vi "Convert Grayscale Image to Binary Image LV2012 NIVerified.vi"() -> ()   [LabVIEW 2021, in "Test VIs.lvclass"]
doc: "This VI demonstrates how to convert a grayscale image into a binary image.\nTo do so, you can use the IMAQ Threshold function with a lower limit = 0 and upper limit = 1."
uses:
  Test VIs/Test VIs.lvclass
  <vilib>/vision/NI_Vision_Development_Module.lvlib
panel:
  in  "Range":cluster{"Lower value":sgl, "Upper value":sgl}={"Lower value"=100.0, "Upper value"=200.0}
  out "Original Image":T1(plugin-control)
  out "Binary Image":T1(plugin-control)
  # "Overview: Demonstrates how to convert a grayscale image into a binary image with the IMAQ Threshold VI. \nRequirements: LabVIEW Base Development System 2012 (or compatible)\n                            NI Vision Development Module 2012 (or compatible)\nInstructions: \n1. Run the VI.\n2. Select a grayscale image which should be converted to a binary image. An example image is already provided with this example."
  # "The palette for this Image Display need to be set to Binary, \notherwise no picture will be displayed.\nRight click on the image and select Palette >> Binary"
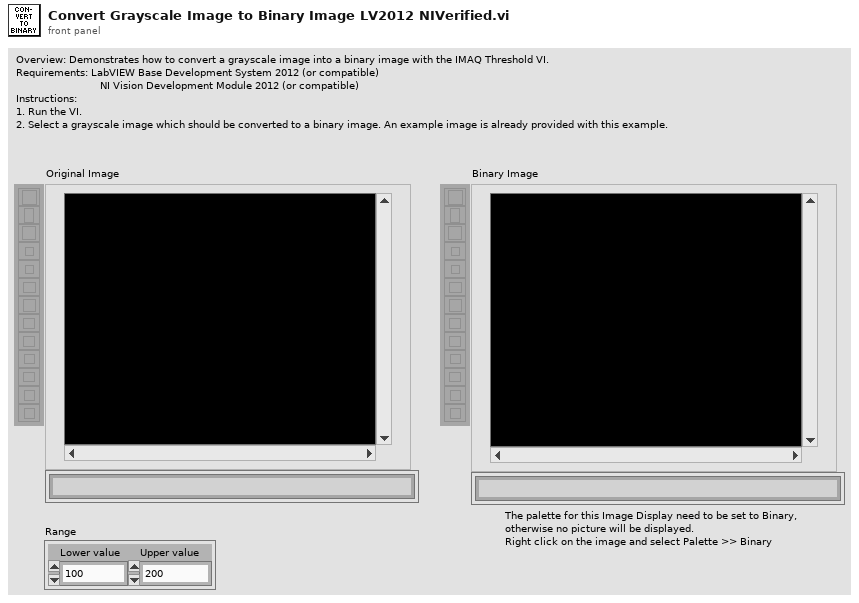
[diagram p1: front panel]
types:
  T1 = typedef "IMAQ Image.ctl" = refnum<image>
  T2 = typedef "Image Type" = u32
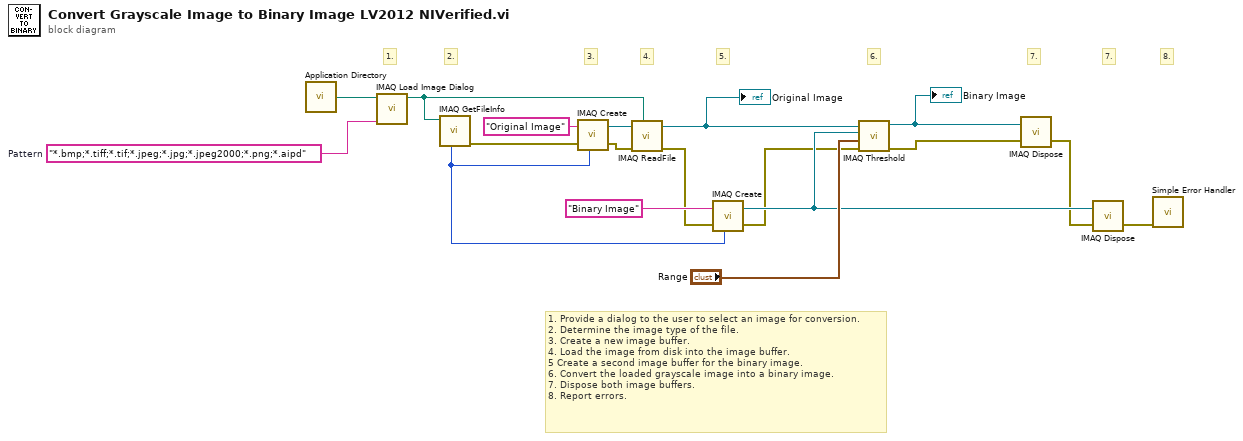
[diagram p0: block diagram]
diagram:
  w10 = "*.bmp;*.tiff;*.tif;*.jpeg;*.jpg;*.jpeg2000;*.png;*.aipd"  # Pattern
  # "8."
  # "7."
  # "7."
  # "6."
  # "5."
  # "4."
  # "3."
  # "2."
  # "1."
  # "1. Provide a dialog to the user to select an image for conversion.\n2. Determine the image type of the file.\n3. Create a new image buffer.\n4. Load the image from disk into the image buffer.\n5 Create a second image buffer for the binary image.\n6. Convert the loaded grayscale image into a binary image.\n7. Dispose both image buffers.\n8. Report errors."
  n1 = call <vilib>:"Application Directory.vi"() -> ("Application Directory"=w1:path)
  n2 = call "IMAQ Load Image Dialog"("Pattern"=w10, "Start Path"=w1) -> ("Path"=w9:path)  [unwired: 7 in, 2 out]
  n3 = call "IMAQ GetFileInfo"("File Path"=w9) -> ("error out"=w7:errorcluster, "Image Type"=w8:T2)  [unwired: 4 in, 5 out]
  n4 = call "IMAQ Create"("Image Name"="Original Image", "Image Type"=w8, "error in (no error)"=w7) -> ("New Image"=w18:T1, "error out"=w16:errorcluster)  [unwired: 2 in]
  n5 = call "IMAQ ReadFile"("File Path"=w9, "error in (no error)"=w16, "Image"=w18) -> ("error out"=w6:errorcluster, "Image Out"=w4:T1)  [unwired: 4 in, 3 out]
  "Original Image" <- w4
  n6 = call "IMAQ Create"("Image Name"="Binary Image", "Image Type"=w8, "error in (no error)"=w6) -> ("New Image"=w13:T1, "error out"=w5:errorcluster)  [unwired: 2 in]
  n7 = call "IMAQ Threshold"("error in (no error)"=w5, "Range"="Range", "Image Dst"=w13, "Image Src"=w4) -> ("error out"=w2:errorcluster, "Image Dst Out"=w3:T1)  [unwired: 6 in]
  "Binary Image" <- w3
  n8 = call "IMAQ Dispose"("Image"=w3, "error in (no error)"=w2) -> ("error out"=w12:errorcluster)  [unwired: 4 in]
  n9 = call "IMAQ Dispose"("Image"=w13, "error in (no error)"=w12) -> ("error out"=w11:errorcluster)  [unwired: 4 in]
  n10 = call <vilib>:"Simple Error Handler.vi"("error in (no error)"=w11) -> ()  [unwired: 4 in, 5 out]
